vi "action.vi"(0 "HGF_FGV_Append":refnum<class "HGF_FGV_Delete.lvclass">, 2 "Objects":refnum<class>[](array[class]), 5 "error in (no error)":errorcluster) -> (14 "dup HGF_FGV_Append":refnum<class "HGF_FGV_Delete.lvclass">, 16 "dup Objects":refnum<class>[](array[class]), 19 "error out":errorcluster)   [LabVIEW 2012, in "HGF_FGV.lvlib" / "HGF_FGV_Delete.lvclass"]
doc: "Delete objects from object array."
uses:
  HGF_FGV_Delete.lvclass
  HGF_FGV_Delete.lvclass/HGF_FGV_Delete.ctl
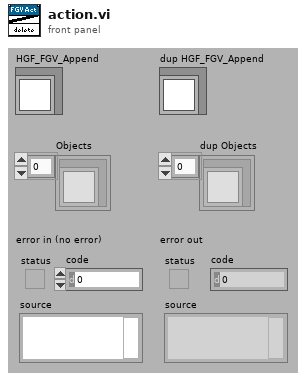
[diagram p1: front panel]
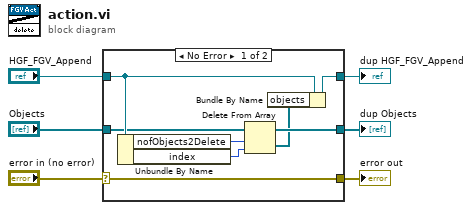
[diagram p0: block diagram]
diagram:
  n1 = case shown="No Error" "error in (no error)" {
    selector: "error in (no error)" -> [w14 w17]
    tunnel: [w14 w17] -> w5
    tunnel: [w13 w16] -> w3
    tunnel: "HGF_FGV_Append" -> [w12 w16]
    tunnel: [w10 w15] -> w2
    tunnel: "Objects" -> [w11 w15]
    frame No Error {
      n2 = Unbundle By Name(w12) -> ("nofObjects2Delete"=w8:u32, "index"=w7:u32)
      n3 = Delete From Array(array=w11, length=w8, index=w7) -> (deleted portion=w9:refnum<class>[], array with subset deleted=w10:refnum<class>[])
      n4 = Bundle By Name(cluster=w12, "objects"=w9) -> (w13:refnum<class "HGF_FGV_Delete.lvclass">)
    }
    frame Error {
    }
  }
  "error out" <- w5
  "dup HGF_FGV_Append" <- w3
  "dup Objects" <- w2
